vi "Connection Status.vi"(8 "error in (no error)":errorcluster, 9 "Remarks":string, 10 "Status":bool, 11 "Controller in":refnum<class "Controller.lvclass">) -> (0 "error out":errorcluster, 3 "Controller out":refnum<class "Controller.lvclass">)   [LabVIEW 2022 SP3, in "Controller.lvlib" / "Controller.lvclass"]
uses:
  Controller.lvclass
  Controller.lvclass/Controller.ctl
  UserInterface/UserInterface Messages/Sensor Status Msg/Sensor Status Msg.lvclass/Sensor Status Msg.ctl
  <vilib>/ActorFramework/Message Enqueuer/Message Enqueuer.lvclass/Message Enqueuer.ctl
  UserInterface/UserInterface Messages/Log Data Msg/Log Data Msg.lvclass/Log Data Msg.ctl
  <vilib>/ActorFramework/Message Enqueuer/Enqueue.vi
  UserInterface/UserInterface Messages/Sensor Status Msg/Sensor Status Msg.lvclass
  C:/Program Files/National Instruments/LabVIEW 2022/vi.lib/ActorFramework/Message/Message.lvclass
  UserInterface/UserInterface Messages/Log Data Msg/Log Data Msg.lvclass
  <vilib>/ActorFramework/Message Priority Queue/Priority Enqueue.vi
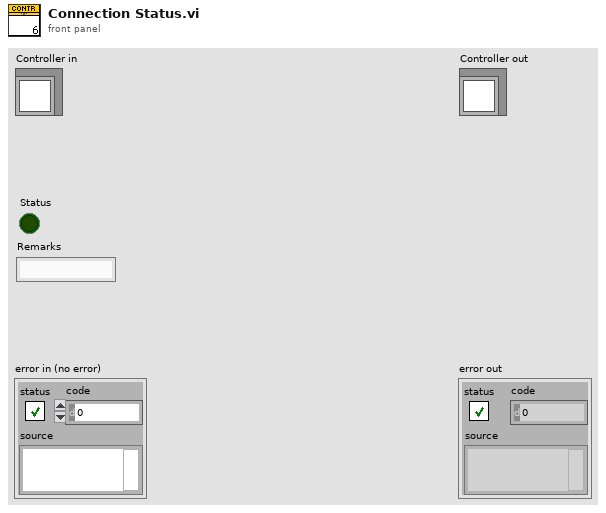
[diagram p1: front panel]
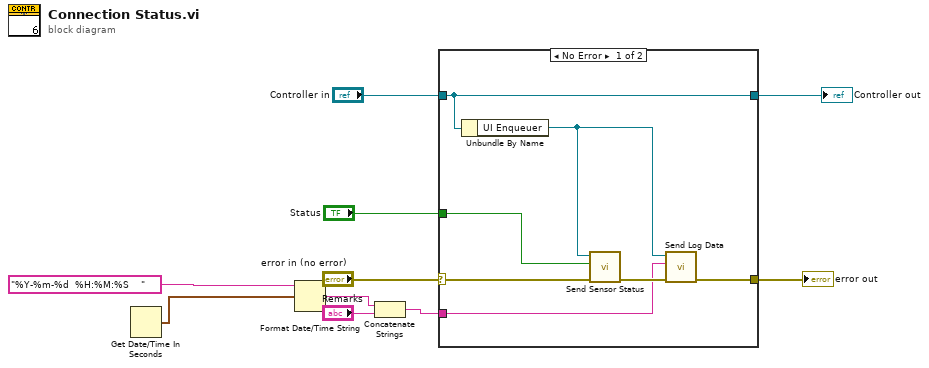
[diagram p0: block diagram]
diagram:
  n1 = Get Date/Time In Seconds() -> (seconds since 1Jan1904=w2:timestamp)
  n2 = Format Date/Time String(time format string (%c)="%Y-%m-%d  %H:%M:%S    ", seconds (now)=w2) -> (date/time string=w1:string)  [unwired: 1 in]
  n3 = Concatenate Strings(w1, "Remarks") -> (w4:string)
  n4 = case shown="No Error" "error in (no error)" {
    selector: "error in (no error)" -> [w17 w18]
    tunnel: "Controller in" -> [w16 w19]
    tunnel: [w16 w19] -> w8
    tunnel: [w12 w18] -> w7
    tunnel: "Status" -> [w15 _]
    tunnel: w4 -> [w11 _]
    frame No Error {
      n5 = Unbundle By Name(w16) -> ("UI Enqueuer"=w14:refnum<class "Message Enqueuer.lvclass">)
      n6 = call "Send Sensor Status.vi"("error in (no error)"=w17, "Sensor Status"=w15, "Message Enqueuer"=w14) -> ("error out"=w13:errorcluster)  [unwired: 7 in, 1 out]
      n7 = call "Send Log Data.vi"("error in (no error)"=w13, "Message"=w11, "Message Enqueuer"=w14) -> ("error out"=w12:errorcluster)  [unwired: 7 in, 1 out]
    }
    frame Error {
    }
  }
  "error out" <- w7
  "Controller out" <- w8
